vi "smu Timed current  Sweep.vi"() -> ()   [LabVIEW 2017]
doc: "Demonstrates how to sweep the voltage on a single channel and display the results in a graph. This example performs a hardware-timed sweep using Sequence source mode."
uses:
  <instrlib>/niDCPower/nidcpower.llb/niDCPower Source Mode.ctl
  <instrlib>/niDCPower/nidcpower.llb/niDCPower Output Function.ctl
panel:
  out "averaged resistance":dbl
  out "averaged current":dbl format="%0.3f"
  out "averaged voltage":dbl format="%0.2f"
  in  "Timeout (Sec)":dbl=10.0 format="%.3p"
  in  "Source Delay (Sec)":dbl=0.005
  in  "Voltage limit":dbl=0.01 caption="Voltage  Limit"
  in  "Channel Name":string="0"
  in  "Current Level End":dbl=5.0 caption="Current Level Stop"
  in  "Current Level Start":dbl=1.0
  in  "Points":i32=10 caption="Points to average" min=1
  in  "Resource Name":refnum<k15>="Dev1"
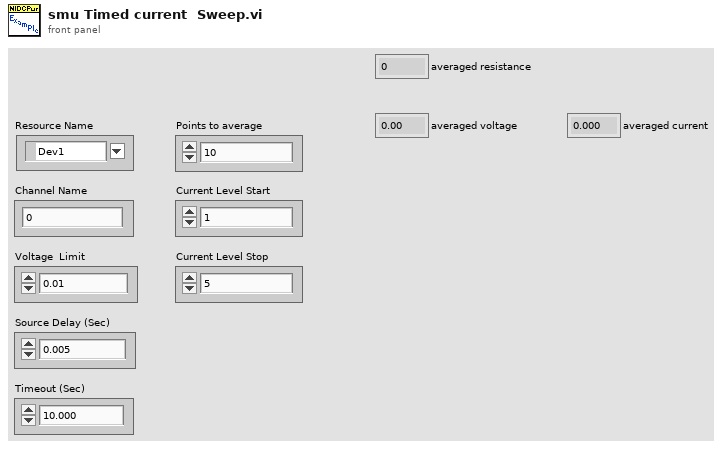
[diagram p1: front panel]
types:
  T1 = typedef "niDCPower Output Function.ctl" = i32
  T2 = typedef "niDCPower Source Mode.ctl" = i32
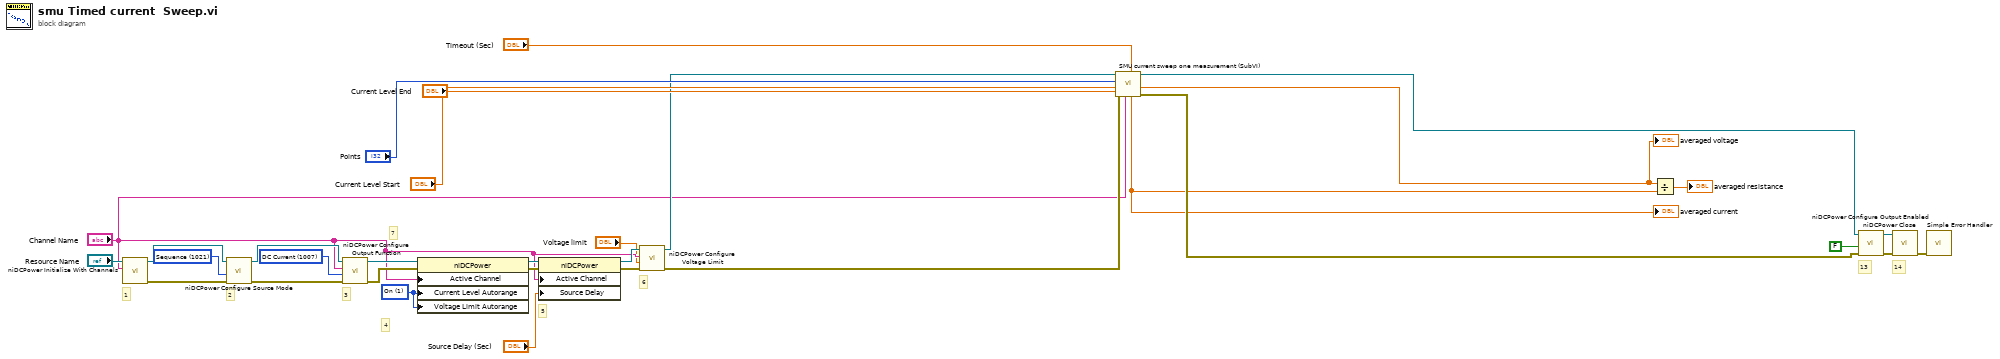
[diagram p0: block diagram]
diagram:
  w11 = T1 1007 items=["DC Voltage"=1006, "DC Current"=1007, "Pulse Voltage"=1049, "Pulse Current"=1050] ("output function")
  w24 = T2 1021 items=["Single Point"=1020, "Sequence"=1021] ("source mode")
  w12 = 1 items=["Off", "On"] ("DC Voltage:Voltage Level Autorange")
  # "6"
  # "7"
  # "5"
  # "2"
  # "14"
  # "13"
  # "4"
  # "3"
  # "1"
  n1 = call <instrlib>:"niDCPower Initialize With Channels.vi"("channels"="Channel Name", "resource name"="Resource Name") -> ("error out"=w28:errorcluster, "instrument handle out"=w25:refnum<k15>)  [unwired: 3 in, 5 out]
  n2 = call <instrlib>:"niDCPower Configure Source Mode.vi"("error in (no error)"=w28, "source mode"=w24, "instrument handle"=w25) -> ("error out"=w27:errorcluster, "instrument handle out"=w26:refnum<k15>)  [unwired: 7 out]
  n3 = call <instrlib>:"niDCPower Configure Output Function.vi"("error in (no error)"=w27, "output function"=w11, "channel name"="Channel Name", "instrument handle"=w26) -> ("error out"=w13:errorcluster, "instrument handle out"=w14:refnum<k15>)  [unwired: 6 out]
  n4 = property class="niDCPower"(reference=w14, error in=w13, "Active Channel"="Channel Name", "Current Level Autorange"=w12, "Voltage Limit Autorange"=w12) -> (reference out=w23:refnum<k15>, error out=w22:errorcluster)
  n5 = property class="niDCPower"(reference=w23, error in=w22, "Active Channel"="Channel Name", "Source Delay"="Source Delay (Sec)") -> (reference out=w4:refnum<k15>, error out=w5:errorcluster)
  n6 = call <instrlib>:"niDCPower Configure Voltage Limit.vi"("error in (no error)"=w5, "voltage limit"="Voltage limit", "channel name"="Channel Name", "instrument handle"=w4) -> ("error out"=w7:errorcluster, "instrument handle out"=w6:refnum<k15>)  [unwired: 6 out]
  n7 = call "SMU current sweep one measurement (SubVI).vi"("Timeout (Sec)"="Timeout (Sec)", "Channel Name"="Channel Name", "Current Level End"="Current Level End", "error in (no error)"=w7, "Current Level Start"="Current Level Start", "Points to average"="Points", "IVI Refnum in"=w6) -> ("error out"=w19:errorcluster, "Average voltage"=w8:dbl, "IVI Refnum out"=w16:refnum<k15>, "Average current"=w9:dbl)  [unwired: 1 in]
  "averaged voltage" <- w8
  "averaged current" <- w9
  n8 = Divide(x=w8, y=w9) -> (x/y=→"averaged resistance":dbl)
  n9 = call <instrlib>:"niDCPower Configure Output Enabled.vi"("error in (no error)"=w19, "output enabled"=FALSE, "instrument handle"=w16) -> ("error out"=w18:errorcluster, "instrument handle out"=w21:refnum<k15>)  [unwired: 1 in, 6 out]
  n10 = call <instrlib>:"niDCPower Close.vi"("error in (no error)"=w18, "instrument handle"=w21) -> ("error out"=w17:errorcluster)  [unwired: 9 out]
  n11 = call <vilib>:"Simple Error Handler.vi"("error in (no error)"=w17) -> ()  [unwired: 1 in, 8 out]
